vi "Table_ChangeTableSortOrder.vi"(8 "error in (no error)":errorcluster, 9 "Column":i32, 10 "State Information in":T1, 11 "Data In":string[][](array[string])) -> (0 "error out":errorcluster, 2 "State Information out":T1, 3 "Data Out":string[][](array[string]))   [LabVIEW 2012, in "TableSupportLib.lvlib"]
uses:
  TableSupportLib.lvlib
  Table_StateInformation.ctl
  Table_ChannelInfoCluster.ctl
  Table_SortArraySettings.ctl
  Table_ListboxSettings.ctl
  <userlib>/_OpenG.lib/array/array.llb/Sort 2D Array (String)__ogtk.vi
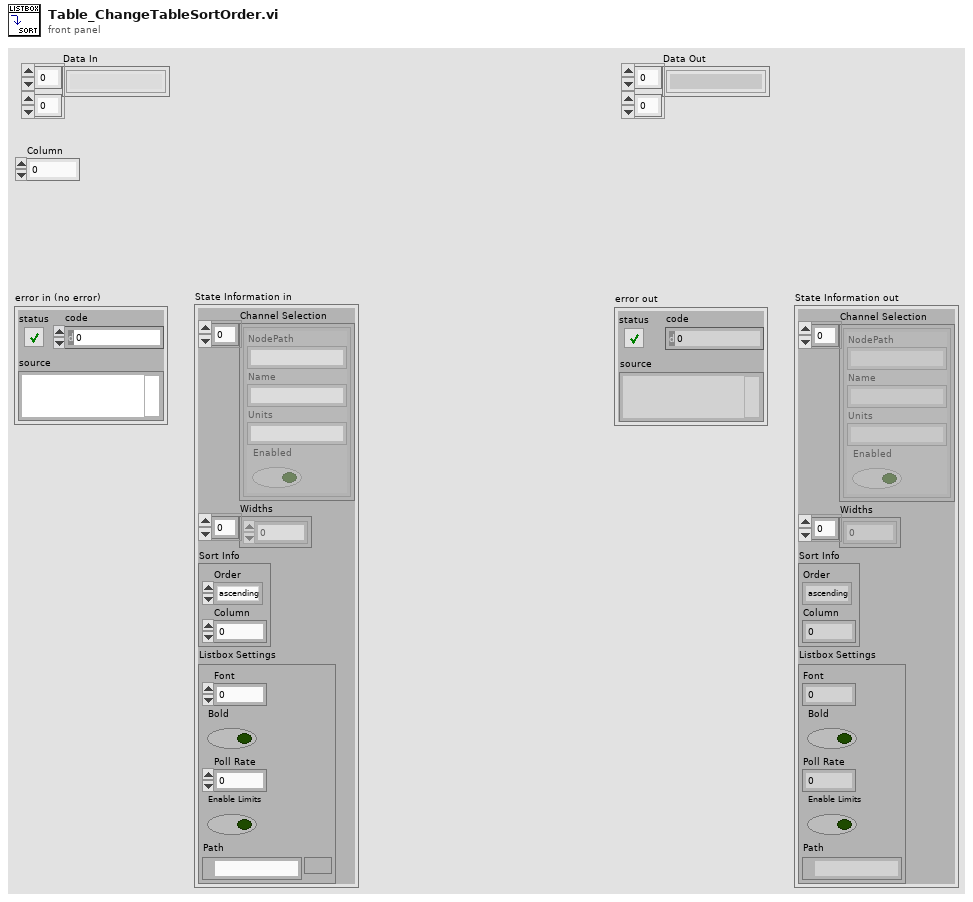
[diagram p1: front panel]
types:
  T1 = typedef "TableSupportLib.lvlib/Table_StateInformation.ctl" = cluster{"Channel Selection":T2[], "Widths":dbl[], "Sort Info":T3, "Listbox Settings":T4}
  T2 = typedef "TableSupportLib.lvlib/Table_ChannelInfoCluster.ctl" = cluster{"NodePath":string, "Name":string, "Units":string, "Enabled":bool}
  T3 = typedef "TableSupportLib.lvlib/Table_SortArraySettings.ctl" = cluster{"Order":enum16{"ascending", "descending"}, "Column":i32}
  T4 = typedef "TableSupportLib.lvlib/Table_ListboxSettings.ctl" = cluster{"Font":u32, "Bold":bool, "Poll Rate":u32, "Enable Limits":bool, "Path":path}
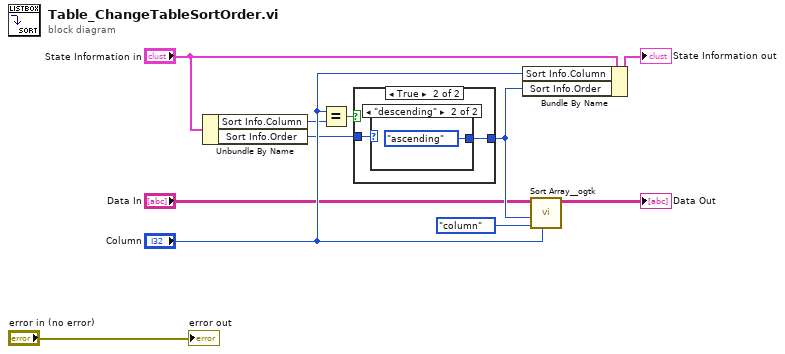
[diagram p0: block diagram]
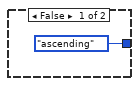
[diagram p2: hidden frame]
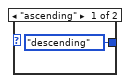
[diagram p3: hidden frame]
diagram:
  n1 = Unbundle By Name("State Information in") -> ("Sort Info.Column"=w4:i32, "Sort Info.Order"=w3:enum16{"ascending", "descending"})
  n2 = Equal?(x="Column", y=w4) -> (x = y?=w5:bool)
  n3 = case shown="True" w5 {
    tunnel: w3 -> [_ w14]
    tunnel: [enum16{"ascending", "descending"}."ascending" ("Order") w13] -> w10
    frame False {
    }
    frame True {
      n4 = case shown="\"descending\"" w14 {
        tunnel: [enum16{"ascending", "descending"}."descending" ("Order") enum16{"ascending", "descending"}."ascending" ("Order")] -> w13
        frame "ascending" {
        }
        frame "descending" {
        }
      }
    }
  }
  n5 = Bundle By Name(cluster="State Information in", "Sort Info.Column"="Column", "Sort Info.Order"=w10) -> (→"State Information out":T1)
  n6 = call-poly <userlib>:"Sort Array__ogtk.vi"("Column/Row to Sort By"="Column", "Sort By in"=enum16{"row", "column"}."column", "Order"=w10, "Array in"="Data In") -> ("Sorted Array out"=→"Data Out":string[][])  [unwired: 4 in, 3 out]
  "error out" <- "error in (no error)"
